vi "TripleCoincidencesCheck.vi"(0 "initialized array":dbl[][](array[numeric]), 1 "Cluster In":T1 {"Coincidence Window" format="%#_13g"; "Delay12" format="%#_13g"; "Delay02" format="%#_13g"; "Delay01" format="%#_13g"}) -> (8 "cluster Out":T1 {"Coincidence Window" format="%#_13g"; "Delay12" format="%#_13g"; "Delay02" format="%#_13g"; "Delay01" format="%#_13g"})   [LabVIEW 2023]
uses:
  Get_Delays_Ctrl.ctl
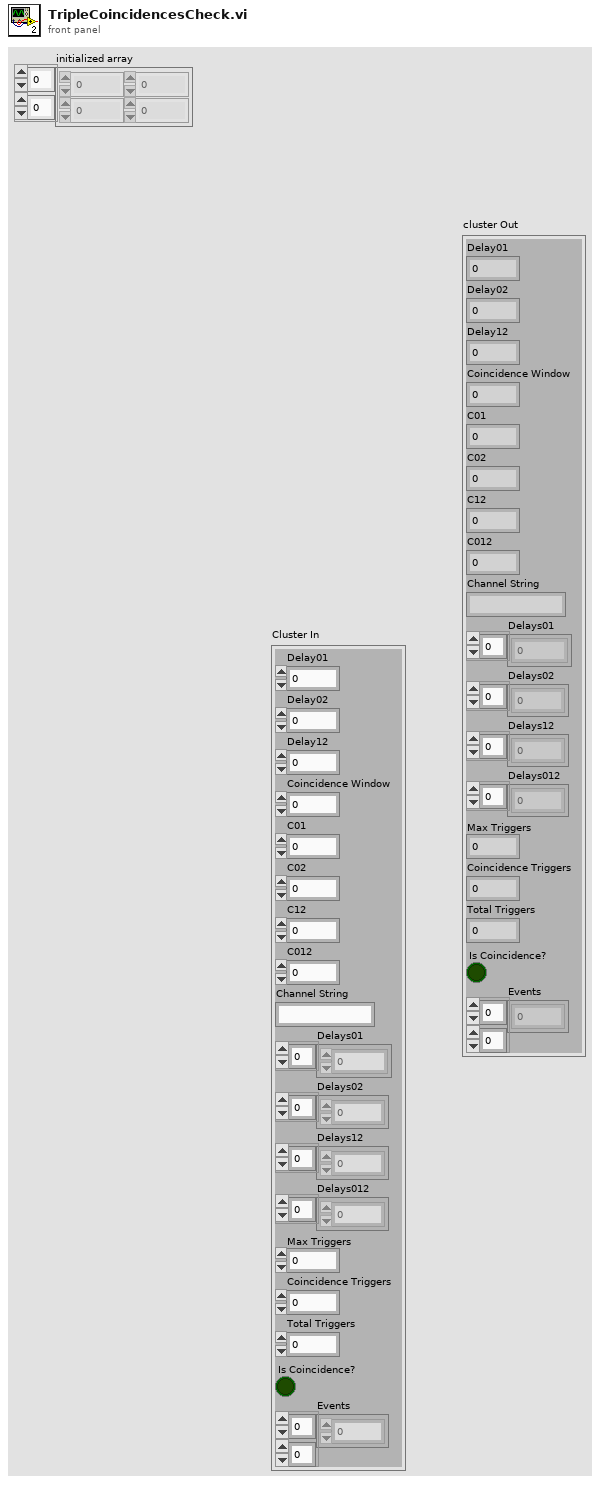
[diagram p1: front panel]
types:
  T1 = typedef "Get_Delays_Ctrl.ctl" = cluster{"Delay01":dbl, "Delay02":dbl, "Delay12":dbl, "Coincidence Window":dbl, "C01":u32, "C02":u32, "C12":u32, "C012":u32, "Channel String":string, "Delays01":sgl[], "Delays02":dbl[], "Delays12":dbl[], "Delays012":dbl[], "Max Triggers":i32, "Coincidence Triggers":i32, "Total Triggers":i32, "Is Coincidence?":bool, "Events":u64[][]}
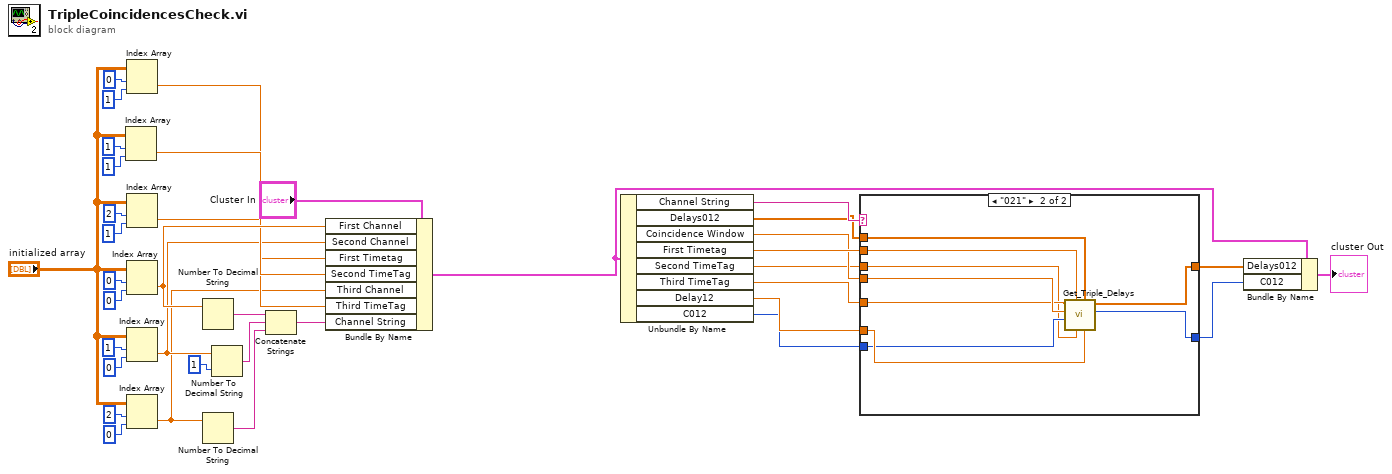
[diagram p0: block diagram]
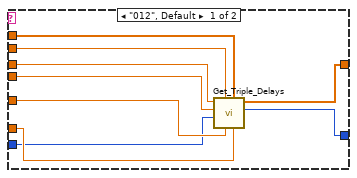
[diagram p2: hidden frame]
diagram:
  n1 = Index Array(array="initialized array", index (row)=1, index (col)=1 ("disabled index (col)")) -> (element=w24:dbl)
  n2 = Index Array(array="initialized array", index (row)=0, index (col)=1 ("disabled index (col)")) -> (element=w23:dbl)
  n3 = Index Array(array="initialized array", index (row)=2, index (col)=1 ("disabled index (col)")) -> (element=w12:dbl)
  n4 = Index Array(array="initialized array", index (row)=0, index (col)=0 ("disabled index (col)")) -> (element=w25:dbl)
  n5 = Index Array(array="initialized array", index (row)=1, index (col)=0 ("disabled index (col)")) -> (element=w22:dbl)
  n6 = Index Array(array="initialized array", index (row)=2, index (col)=0 ("disabled index (col)")) -> (element=w10:dbl)
  n7 = Number To Decimal String(number=w25) -> (decimal integer string=w27:string)  [unwired: 1 in]
  n8 = Number To Decimal String(number=w10) -> (decimal integer string=w9:string)  [unwired: 1 in]
  n9 = Number To Decimal String(number=w22, width (-)=i16 1) -> (decimal integer string=w28:string)
  n10 = Concatenate Strings(w27, w28, w9) -> (w18:string)
  n11 = Bundle By Name(cluster="Cluster In", "First Channel"=w25, "Second Channel"=w22, "First Timetag"=w23, "Second TimeTag"=w24, "Third Channel"=w10, "Third TimeTag"=w12, "Channel String"=w18) -> (w20:T1)
  n12 = Unbundle By Name(w20) -> ("Channel String"=w8:string, "Delays012"=w1:dbl[], "Coincidence Window"=w6:dbl, "First Timetag"=w7:dbl, "Second TimeTag"=w4:dbl, "Third TimeTag"=w5:dbl, "Delay12"=w3:dbl, "C012"=w2:u32)
  n13 = case shown="\"021\"" w8 {
    tunnel: w7 -> [w46 w55]
    tunnel: w6 -> [w42 w53]
    tunnel: w5 -> [w45 w48]
    tunnel: w4 -> [w44 w47]
    tunnel: w3 -> [w43 w54]
    tunnel: w2 -> [w41 w52]
    tunnel: [w40 w51] -> w21
    tunnel: [w39 w50] -> w11
    tunnel: w1 -> [w38 w49]
    frame "012", Default {
      n14 = call "Get_Triple_Delays.vi"("Delay Second-Third"=w43, "Delays012 in"=w38, "Third TimeTag"=w45, "First Timetag"=w46, "C012 in"=w41, "Coincidence Window"=w42, "Second TimeTag"=w44) -> ("C012 out"=w40:u32, "Delays012 out"=w39:dbl[])  [unwired: 3 in]
    }
    frame "021" {
      n15 = call "Get_Triple_Delays.vi"("Delay Second-Third"=w54, "Delays012 in"=w49, "Third TimeTag"=w47, "First Timetag"=w55, "C012 in"=w52, "Coincidence Window"=w53, "Second TimeTag"=w48) -> ("C012 out"=w51:u32, "Delays012 out"=w50:dbl[])  [unwired: 3 in]
    }
  }
  n16 = Bundle By Name(cluster=w20, "Delays012"=w11, "C012"=w21) -> (→"cluster Out":T1)
